vi "TrajectoryUtil_fromPathWeaverJSON.vi"(8 "error in (no error)":errorcluster, 11 "FileName":string="trajectory.json") -> (0 "error out":errorcluster, 3 "outTRAJECTORY":T1 {"TotalTImeSecs" format="%20.3f"})   [LabVIEW 2019, in "Trajectory_Library.lvlib"]
doc: "Imports a Trajectory from a PathWeaver-style JSON file.\n\nParameters:\n - FileName - File name string of the json file to import from\n - Error In - Error cluster (not used)\n\nReturns:\n - Trajectory - Trajectory data structure\n - Error out - Returned error cluster"
uses:
  Trajectory_Library.lvlib
  TRAJECTORY.ctl
  TRAJ_STATE.ctl
  POSE2D.ctl
  TRANSLATION2D.ctl
  ROTATION2D.ctl
  Rotation_CreateAngle.vi
  Translation_Create.vi
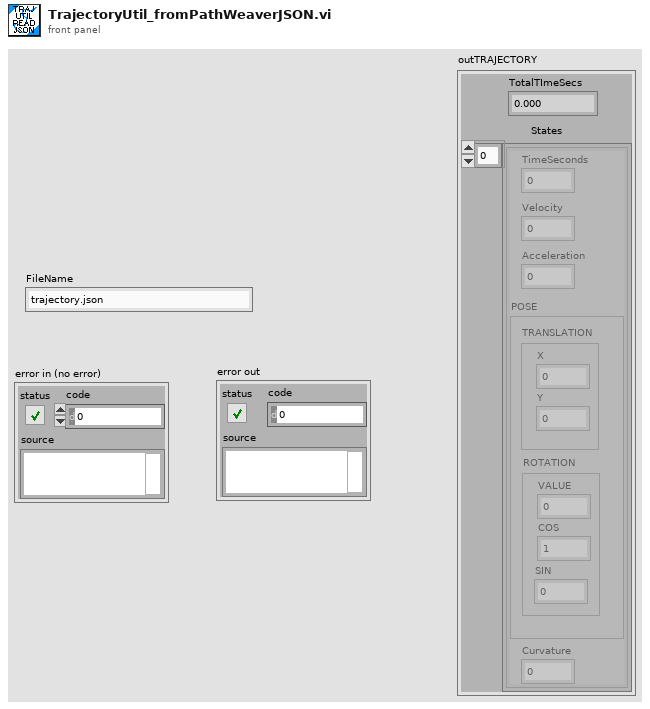
[diagram p1: front panel]
types:
  T1 = typedef "Trajectory_Library.lvlib/TRAJECTORY.ctl" = cluster{"TotalTImeSecs":dbl, "States":T2[]}
  T2 = typedef "Trajectory_Library.lvlib/TRAJ_STATE.ctl" = cluster{"TimeSeconds":dbl, "Velocity":dbl, "Acceleration":dbl, "POSE":T3, "Curvature":dbl}
  T3 = typedef "Trajectory_Library.lvlib/POSE2D.ctl" = cluster{"TRANSLATION":T4, "ROTATION":T5}
  T4 = typedef "Trajectory_Library.lvlib/TRANSLATION2D.ctl" = cluster{"X":dbl, "Y":dbl}
  T5 = typedef "Trajectory_Library.lvlib/ROTATION2D.ctl" = cluster{"VALUE":dbl, "COS":dbl, "SIN":dbl}
  T6 = enum16{"open", "replace", "create", "open or create", "replace or create", "replace or create with confirmation"}
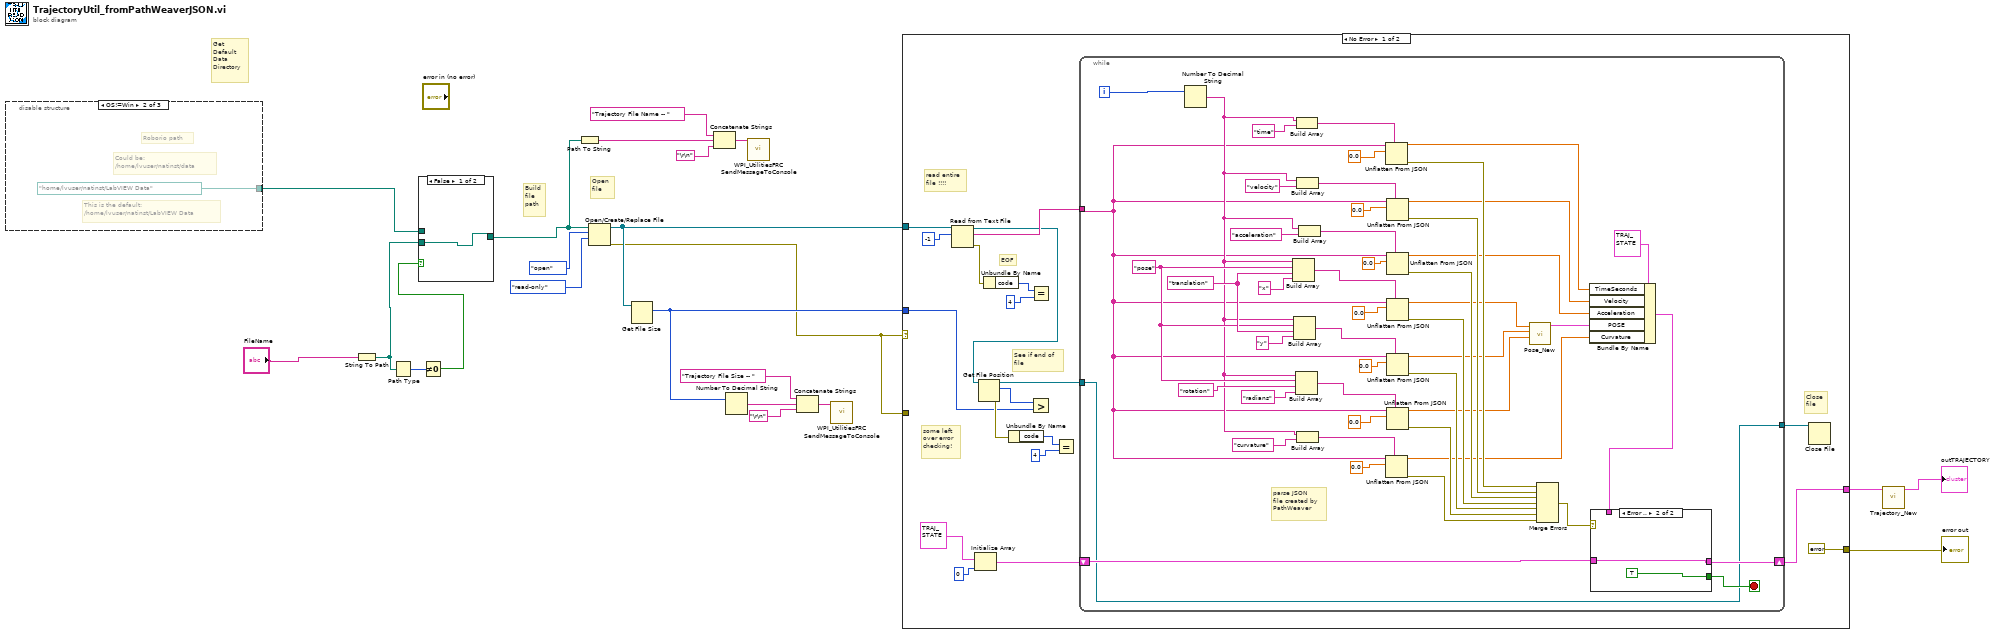
[diagram p0: block diagram]
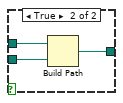
[diagram p2: hidden frame]
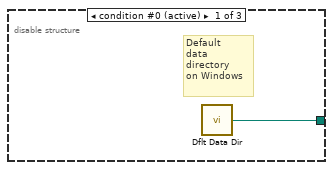
[diagram p3: hidden frame]
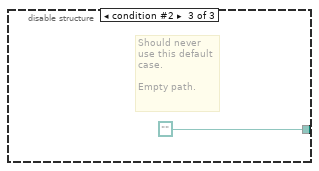
[diagram p4: hidden frame]
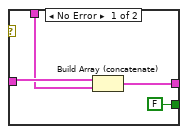
[diagram p5: hidden frame]
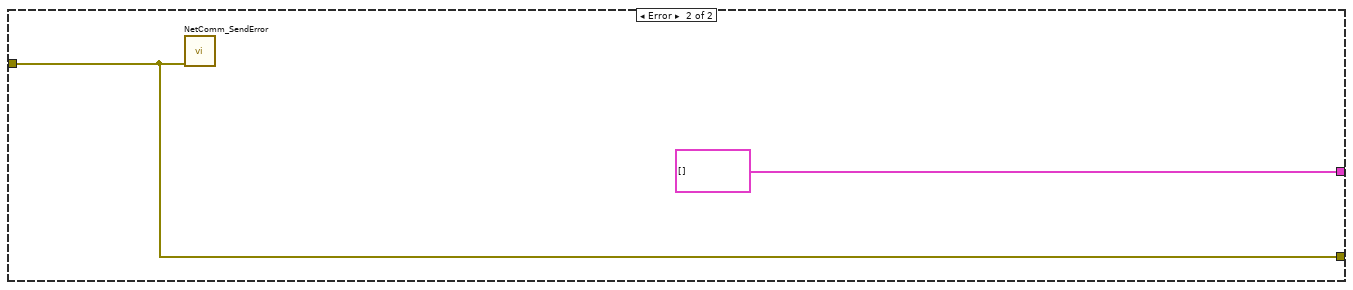
[diagram p6: hidden frame]
diagram:
  # "Get\nDefault\nData\nDirectory"
  # "Open\nfile"
  # "Build\nfile\npath"
  n1 = disable-structure shown="OS!=Win" {
    disable-tunnel: [w23 path "/home/lvuser/natinst/LabVIEW Data" path ""] -> w8
    frame condition #0 (active) {
      # "Default\ndata\ndirectory\non Windows"
      n2 = call <vilib>:"Dflt Data Dir.vi"() -> ("App:Default Data Directory"=w23:path)
    }
    frame condition #1 {
      # "This is the default:\n/home/lvuser/natinst/LabVIEW Data"
      # "Could be:\n/home/lvuser/natinst/data"
      # "Roborio path"
    }
    frame condition #2 {
      # "Should never\nuse this default\ncase.\n\nEmpty path."
    }
  }
  n3 = String To Path(string="FileName") -> (path=w3:path)
  n4 = Path Type(1:w3) -> (0:w2:i16)
  n5 = Not Equal To 0?(x=w2) -> (x != 0?=w1:bool)
  n6 = case shown="False" w1 {
    tunnel: [w26 w29] -> w19
    tunnel: w8 -> [_ w28]
    tunnel: w3 -> [w26 w27]
    frame False {
    }
    frame True {
      n7 = Build Path(base path=w28, name or relative path=w27) -> (appended path=w29:path)
    }
  }
  n8 = Path To String(path=w19) -> (string=w12:string)
  n9 = Open/Create/Replace File(file path (use dialog)=w19, operation (0:open)=T6."open", access (0:read/write)=enum16{"read/write", "read-only", "write-only"}."read-only") -> (refnum out=w20:refnum<file>, error out=w9:errorcluster)  [unwired: 3 in, 1 out]
  n10 = Get File Size(file=w20) -> (size (in bytes)=w15:i64)  [unwired: 1 in, 2 out]
  n11 = Concatenate Strings("Trajectory File Name -- ", w12, "\r\n") -> (w10:string)
  n12 = Number To Decimal String(number=w15) -> (decimal integer string=w16:string)  [unwired: 1 in]
  n13 = call <vilib>:"WPI_UtilitiesFRC SendMessageToConsole.vi"("Message"=w10) -> ()  [unwired: 14 in, 1 out]
  n14 = Concatenate Strings("Trajectory File Size -- ", w16, "\r\n") -> (w18:string)
  n15 = call <vilib>:"WPI_UtilitiesFRC SendMessageToConsole.vi"("Message"=w18) -> ()  [unwired: 14 in, 1 out]
  n16 = case shown="No Error" w9 {
    tunnel: w20 -> [w42 _]
    tunnel: w15 -> [w33 _]
    tunnel: [w46 T2[] []] -> w7
    tunnel: w9 -> [_ w104]
    tunnel: [errorcluster {"status"=FALSE, "code"=0, "source"=""} ("error out") w104] -> w5
    frame No Error {
      # "some left\nover error\nchecking!"
      # "See if end of \nfile"
      # "EOF"
      # "read entire\nfile !!!!"
      # "Close\nfile"
      n17 = Read from Text File(file (use dialog)=w42, count=-1) -> (refnum out=w32:refnum<file>, text=w41:string, error out=w38:errorcluster)  [unwired: 2 in, 1 out]
      n18 = Initialize Array(T2 {"TimeSeconds"=0.0, "Velocity"=0.0, "Acceleration"=0.0, "POSE"={"TRANSLATION"={"X"=0.0, "Y"=0.0}, "ROTATION"={"VALUE"=0.0, "COS"=1.0, "SIN"=0.0}}, "Curvature"=0.0} ("TRAJ_STATE"), 0 ("dimension size")) -> (w47:T2[])
      n19 = Get File Position(7:w32) -> (0:w37:errorcluster, 2:w35:i64, 3:w31:refnum<file>)  [unwired: 1 in]
      n20 = Unbundle By Name(w38) -> ("code"=w40:i32)
      n21 = Unbundle By Name(w37) -> ("code"=w36:i32)
      n22 = Greater?(x=w35, y=w33) -> ()  [unwired: 1 out]
      n23 = Equal?(x=w40, y=4) -> ()  [unwired: 1 out]
      n24 = Equal?(x=w36, y=4) -> ()  [unwired: 1 out]
      n25 = while {
        shift-right: [w97] -> w46
        shift-left: w47 -> [w50]
        tunnel: w41 -> [w51]
        tunnel: w31 -> [w49]
        tunnel: [w49] -> w30
        i -> [w53]
        stop <- w54 stop-if-true
        w66 = "translation"
        w64 = "pose"
        # "parse JSON\nfile created by\nPathWeaver"
        n26 = Number To Decimal String(number=w53) -> (decimal integer string=w52:string)  [unwired: 1 in]
        n27 = Build Array(w52, w64, w66, "x") -> (w62:string[])
        n28 = Build Array(w52, w64, w66, "y") -> (w61:string[])
        n29 = Build Array(w52, w64, "rotation", "radians") -> (w60:string[])
        n30 = Build Array(w52, "time") -> (w72:string[])
        n31 = Build Array(w52, "velocity") -> (w69:string[])
        n32 = Build Array(w52, "curvature") -> (w57:string[])
        n33 = Build Array(w52, "acceleration") -> (w68:string[])
        n34 = Unflatten From JSON(path=w72, JSON string=w51, type and defaults=0.0) -> (value=w86:dbl, error out=w95:errorcluster)  [unwired: 4 in]
        n35 = Unflatten From JSON(path=w57, JSON string=w51, type and defaults=0.0) -> (value=w74:dbl, error out=w79:errorcluster)  [unwired: 4 in]
        n36 = Unflatten From JSON(path=w69, JSON string=w51, type and defaults=0.0) -> (value=w85:dbl, error out=w94:errorcluster)  [unwired: 4 in]
        n37 = Unflatten From JSON(path=w68, JSON string=w51, type and defaults=0.0) -> (value=w84:dbl, error out=w93:errorcluster)  [unwired: 4 in]
        n38 = Unflatten From JSON(path=w62, JSON string=w51, type and defaults=0.0) -> (value=w78:dbl, error out=w92:errorcluster)  [unwired: 4 in]
        n39 = Unflatten From JSON(path=w61, JSON string=w51, type and defaults=0.0) -> (value=w77:dbl, error out=w91:errorcluster)  [unwired: 4 in]
        n40 = Unflatten From JSON(path=w60, JSON string=w51, type and defaults=0.0) -> (value=w76:dbl, error out=w90:errorcluster)  [unwired: 4 in]
        n41 = call "Pose_New.vi"("Heading"=w76, "Y"=w77, "X"=w78) -> ("out POSe"=w75:T3)  [unwired: 8 in]
        n42 = Merge Errors(w95, w94, w93, w92, w91, w90, w79) -> (w56:errorcluster)
        n43 = Bundle By Name(cluster=T2 {"TimeSeconds"=0.0, "Velocity"=0.0, "Acceleration"=0.0, "POSE"={"TRANSLATION"={"X"=0.0, "Y"=0.0}, "ROTATION"={"VALUE"=0.0, "COS"=1.0, "SIN"=0.0}}, "Curvature"=0.0} ("TRAJ_STATE"), "TimeSeconds"=w86, "Velocity"=w85, "Acceleration"=w84, "POSE"=w75, "Curvature"=w74) -> (w55:T2)
        n44 = case shown="Error .." w56 {
          tunnel: [FALSE TRUE] -> w54
          tunnel: w50 -> [w100 w102]
          tunnel: w55 -> [w99 _]
          tunnel: [w98 w102] -> w97
          frame No Error {
            n45 = Build Array (concatenate)(w100, w99) -> (w98:T2[])
          }
          frame Error {
          }
        }
      }
      n46 = Close File(refnum=w30) -> ()  [unwired: 1 in, 2 out]
    }
    frame Error {
      n47 = call <vilib>:"NetComm_SendError.vi"("error in (no error)"=w104) -> ()  [unwired: 11 in]
    }
  }
  "error out" <- w5
  n48 = call "Trajectory_New.vi"("TRAJ_STATES"=w7) -> ("TRAJECTORY"=→"outTRAJECTORY":T1)  [unwired: 10 in]
